vi "Diagnostics Main.vi"() -> ()   [LabVIEW 2015, in "Diagnostics Addon Engine.lvlib"]
uses:
  Diagnostics Addon Engine.lvlib
  Types/Main Configuration.ctl
  Shared/Types/Section Properties.ctl
  Shared/Types/CAN Configuration.ctl
  Shared/Types/CAN Interface.ctl
  Shared/Types/Diagnostic Protocols.ctl
  Shared/Types/Transport Protocols.ctl
  Shared/Types/Security.ctl
  Shared/Types/FPGA Bitfile Settings.ctl
  Shared/Types/Frame Parameters.ctl
  Shared/Types/Signal Parameters.ctl
  Shared/Types/DPID Parameters.ctl
  Shared/Types/DPID Periodic Rate.ctl
  <vilib>/Automotive Diagnostic Command Set/Diagnostic Protocols.llb/DTC Descriptor.ctl
  Types/VS Data Channels.ctl
  SubVIs/Inline Async API/Controls/Write To VS Engine.ctl
  <vilib>/NI Veristand/Custom Device API/Data Reference.ctl
  SubVIs/Inline Async API/Controls/Read From VS Engine.ctl
  <vilib>/NI Veristand/Custom Device API/Block Data Reference.ctl
  SubVIs/Inline Async API/Controls/ReadWrite Data.ctl
  SubVIs/Stop FG/Stop Global Commands.ctl
  SubVIs/Initialize TCP Refs.vi
  STM/RQST Comm_Close All Connections.vi
  SubVIs/Cleanup Conversion Sessions.vi
  STM/RQST Comm Lookup Table_Actions.vi
  <vilib>/Utility/error.llb/Clear Errors.vi
  STM/TCP/STM Get Connection Reference (TCP).vi
  SubVIs/Read GMLAN PIDs and DTCs.vi
  SubVIs/UDS Diagnostics Engine.vi
  <vilib>/NI/Tools/Keyed Array/Add.vi
  <vilib>/NI/AMC/Send Local Message.vi
  <vilib>/NI/AMC/Read Next Message.vi
  STM/TCP Check Connection.vi
  <vilib>/NI/AMC/Send Local Messages.vi
  SubVIs/ScaleAndReplaceAcquiredData.vi
  SubVIs/Initialize Raw XNET Frame.vi
  SubVIs/GMLAN/Utilities/Convert Data to DTCs.vi
  SubVIs/Determine Active DTCs and Timestamps.vi
  SubVIs/Convert Boolean to DBL Array.vi
  SubVIs/GMLAN/_SubVIs/ReadDiagnosticInformation_ByStatus.vi
  SubVIs/GMLAN/_SubVIs/ReadDiagnosticInformation_sendOnChangeDTCCount.vi
  SubVIs/GMLAN/_SubVIs/ReadDiagnosticInformation_readStatusOfDTCByDTCNumber.vi
  SubVIs/GMLAN/_SubVIs/ReadFailureRecordData_readFailureRecordParameters.vi
  SubVIs/GMLAN/GMLAN DynamicallyDefineMessage.vi
  SubVIs/GMLAN/GMLAN ReadDataByPacketIdentifier.vi
  SubVIs/GMLAN/GMLAN InitiateDiagnosticOperation.vi
  SubVIs/GMLAN/GMLAN DisableNormalCommunication.vi
  SubVIs/GMLAN/GMLAN ReturnToNormalMode.vi
  SubVIs/Unlock ECU Security.vi
  <vilib>/NI/Tools/Keyed Array/Index.vi
  SubVIs/GMLAN/GMLAN ClearDiagnosticInformation.vi
  SubVIs/GMLAN/GMLAN DeviceControl.vi
  SubVIs/IndexAndScaleGeneratedData.vi
  SubVIs/GMLAN/GMLAN ReadDataByParameterIdentifier.vi
  SubVIs/Read PIDDIDs.vi
  SubVIs/Tester Present.vi
  <vilib>/NI/Tools/Keyed Array/Map String.vi
  <vilib>/NI/AMC/Create Single Message.vi
  <vilib>/NI/AMC/Update Message Routing Info.vi
  <vilib>/NI/AMC/Read Termination Message.vi
  <vilib>/NI/AMC/Create Multiple Messages.vi
  SubVIs/GMLAN/Utilities/Convert Raw Data to DTCs.vi
  SubVIs/GMLAN/Utilities/GMLAN Service Broadcast.vi
  SubVIs/Execute Security DLL.vi
  SubVIs/GMLAN/GMLAN SecurityAccess.vi
  SubVIs/GMLAN/_SubVIs/SecurityAccess_sendKey.vi
  SubVIs/GMLAN/_SubVIs/SecurityAccess_requestSeed.vi
  SubVIs/GMLAN/GMLAN ReadDataByIdentifier.vi
  SubVIs/GMLAN/GMLAN TesterPresent.vi
  <vilib>/NI/Tools/String/Get Case Matching.vi
  <vilib>/NI/AMC/Destroy Message Queue.vi
  <vilib>/Automotive Diagnostic Command Set/Diagnostic Transport.llb/Close Diagnostic.vi
  <vilib>/xnet/xnet.llb/XNET Database Close.vi
  <vilib>/xnet/xnet.llb/XNET Database Close (Database).vi
  <vilib>/xnet/xnet.llb/XNET Database Delete Object.vi
  <vilib>/xnet/xnet.llb/XNET Database Delete (Cluster).vi
  <vilib>/xnet/xnet.llb/XNET Clear.vi
  Shared/SubVIs/GUID Lookup.vi
  STM/Clear Specific Error.vi
  STM/STM Read Meta Data.vi
  STM/TCP/STM Read Meta Data (TCP Ref).vi
  <vilib>/NI/AMC/Send Message.vi
  <vilib>/Automotive Diagnostic Command Set/Diagnostic Protocols.llb/Convert to Phys.vi
  <vilib>/xnet/xnet.llb/XNET Convert.vi
  <vilib>/xnet/xnet.llb/XNET Convert (Frame Raw to Signal).vi
  SubVIs/Convert ID to Raw Data.vi
  <vilib>/xnet/xnet.llb/XNET Read.vi
  <vilib>/xnet/xnet.llb/XNET Read (Frame CAN).vi
  <vilib>/NI/AMC/Globals.vi
  <vilib>/Automotive Diagnostic Command Set/Diagnostic Protocols.llb/UDS TesterPresent.vi
  <vilib>/Automotive Diagnostic Command Set/Diagnostic Transport.llb/Apply Success Failure Error.vi
  <vilib>/Automotive Diagnostic Command Set/Diagnostic Transport.llb/Diagnostic Service.vi
  <vilib>/Automotive Diagnostic Command Set/Diagnostic Transport.llb/Apply Diagnostic Error.vi
  <vilib>/Automotive Diagnostic Command Set/Diagnostic Transport.llb/Diagnostic Response Recv.vi
  <vilib>/Automotive Diagnostic Command Set/Diagnostic Transport.llb/Diagnostic Service Send.vi
  <vilib>/Automotive Diagnostic Command Set/Diagnostic Transport.llb/Diag Globals.vi
  <vilib>/Automotive Diagnostic Command Set/Diagnostic Protocols.llb/TesterPresent.vi
  <vilib>/Automotive Diagnostic Command Set/Diagnostic Protocols.llb/UDS RoutineControl.vi
  <vilib>/Automotive Diagnostic Command Set/Diagnostic Protocols.llb/StopRoutineByLocalIdentifier.vi
  <vilib>/xnet/xnet.llb/XNET Convert (Signal to Frame Raw).vi
  <vilib>/Automotive Diagnostic Command Set/Diagnostic Protocols.llb/RequestRoutineResultsByLocalIdentifier.vi
  <vilib>/Automotive Diagnostic Command Set/Diagnostic Protocols.llb/StartRoutineByLocalIdentifier.vi
  <vilib>/Automotive Diagnostic Command Set/Diagnostic Protocols.llb/UDS InputOutputControlByIdentifier.vi
  <vilib>/Automotive Diagnostic Command Set/Diagnostic Protocols.llb/InputOutputControlByLocalIdentifier.vi
  <vilib>/Automotive Diagnostic Command Set/Diagnostic Protocols.llb/UDS WriteDataByIdentifier.vi
  <vilib>/Automotive Diagnostic Command Set/Diagnostic Protocols.llb/WriteMemoryByAddress.vi
  <vilib>/Automotive Diagnostic Command Set/Diagnostic Protocols.llb/UDS ReadDataByIdentifier.vi
  <vilib>/Automotive Diagnostic Command Set/Diagnostic Protocols.llb/ReadMemoryByAddress.vi
  <vilib>/Automotive Diagnostic Command Set/Diagnostic Protocols.llb/UDS ECUReset.vi
  <vilib>/Automotive Diagnostic Command Set/Diagnostic Protocols.llb/ECUReset.vi
  <vilib>/Automotive Diagnostic Command Set/Diagnostic Protocols.llb/ReadDataByLocalIdentifier.vi
  <vilib>/Automotive Diagnostic Command Set/Diagnostic Protocols.llb/WriteDataByLocalIdentifier.vi
  <vilib>/Automotive Diagnostic Command Set/Diagnostic Protocols.llb/UDS ClearDiagnosticInformation.vi
  <vilib>/Automotive Diagnostic Command Set/Diagnostic Protocols.llb/ClearDiagnosticInformation.vi
  <vilib>/Automotive Diagnostic Command Set/Diagnostic Protocols.llb/ControlDTCSetting.vi
  <vilib>/Automotive Diagnostic Command Set/Diagnostic Protocols.llb/UDS ControlDTCSetting.vi
  <vilib>/Automotive Diagnostic Command Set/Diagnostic Protocols.llb/ReadDTCByStatus.vi
  <vilib>/Automotive Diagnostic Command Set/Diagnostic Protocols.llb/ReadStatusOfDTC.vi
  <vilib>/Automotive Diagnostic Command Set/Diagnostic Protocols.llb/UDS ReportDTCByStatusMask.vi
  <vilib>/Automotive Diagnostic Command Set/Diagnostic Protocols.llb/UDS ReportSeverityInformationOfDTC.vi
  <vilib>/Automotive Diagnostic Command Set/Diagnostic Protocols.llb/UDS ReportDTCBySeverityMaskRecord.vi
  <vilib>/Automotive Diagnostic Command Set/Diagnostic Protocols.llb/SendKey.vi
  <vilib>/Automotive Diagnostic Command Set/Diagnostic Protocols.llb/UDS SendKey.vi
  <vilib>/Automotive Diagnostic Command Set/Diagnostic Protocols.llb/RequestSeed.vi
  <vilib>/Automotive Diagnostic Command Set/Diagnostic Protocols.llb/UDS RequestSeed.vi
  <vilib>/Automotive Diagnostic Command Set/Diagnostic Protocols.llb/EnableNormalMessageTransmission.vi
  <vilib>/Automotive Diagnostic Command Set/Diagnostic Protocols.llb/UDS CommunicationControl.vi
  <vilib>/Automotive Diagnostic Command Set/Diagnostic Protocols.llb/DisableNormalMessageTransmission.vi
  <vilib>/Automotive Diagnostic Command Set/Diagnostic Protocols.llb/UDS DiagnosticSessionControl.vi
  <vilib>/Automotive Diagnostic Command Set/Diagnostic Protocols.llb/StopDiagnosticSession.vi
  <vilib>/Automotive Diagnostic Command Set/Diagnostic Protocols.llb/StartDiagnosticSession.vi
  <vilib>/Automotive Diagnostic Command Set/Diagnostic Transport.llb/Diag Set Property.vi
  <vilib>/Automotive Diagnostic Command Set/Diagnostic Transport.llb/Diag Get Property.vi
  SubVIs/Sort DPID IDs by Speed.vi
  STM/TCP/STM Write Message (TCP).vi
  <vilib>/NI/AMC/Create Message Queue.vi
  STM/TCP/STM Read Message (TCP).vi
  SubVIs/Stop FG/Initialize Global Stop.vi
  SubVIs/Initialize CAN.vi
  STM/RQST Comm Lookup Table_Initialize.vi
  SubVIs/Stop FG/Stop FG.lvlib
  <vilib>/NI Veristand/Custom Device Tools/Custom Device Utility Library/Custom Device Utility Library.lvlib
  SubVIs/Inline Async API/Inline Async API.lvlib
  SubVIs/Error Handling API/Error Handling API.lvlib
  <vilib>/Utility/error.llb/DialogType.ctl
  Shared/Diagnostics Addon Shared.lvlib
  <vilib>/NI Veristand/Custom Device API/Custom Device API.lvlib
panel:
  in  "Parameters":T1={"Properties"={"Name"="", "CAN"={"Database File"=path "", "CAN Interface"=enum."CAN0", "Baud Rate"=0, "Diagnostic Protocol"=enum."GMLAN", "Transport Protocol"=enum."ISO TP - Normal Mode", "Transmit ID"=0, "Receive ID"=0, "Transmit Extension"=0, "Receive Extension"=0, "Receive UUDT ID"=0, "Enable Stream"=TRUE, "VW TP Channel ID"=0, "Security"={"Source DLL Path"=path "", "Security Level"=1, "Target DLL Path"=path ""}, "Fill Frame"=FALSE, "Fill Byte"=255, "Termination"=FALSE}, "FPGA Settings"={"RT Bitfile Path"=path "", "RIO Device"=0, "Enable"=FALSE}, "PIDs"=[], "PID Lookup"=variant, "CPIDs"=[], "CPID Lookup"=variant, "DIDs"=[], "DID Lookup"=variant, "DPIDs"=[], "DPID Lookup"=variant, "DTC descriptor"={"DTC Byte Length"=2, "Status Byte Length"=1, "Add Data Byte Length"=1, "Byte Order"=enum."Motorola"}, "Routine.Start.Cmd Lookup"=variant, "Routine.Status.Cmd Lookup"=variant, "Routine.Stop.Cmd Lookup"=variant, "IO.Cmd Lookup"=variant, "IO.Resp Lookup"=variant, "Routine.Start.Resp Lookup"=variant, "Routine.Status.Resp Lookup"=variant, "Routine.Stop.Resp Lookup"=variant, "Memory.Write Lookup"=variant, "Memory.Read Lookup"=variant}, "ChanRefs"={"ToVS.PIDs"={"Name"="", "Write to VS Engine FIFO"=refnum, "Pairs"={"Refs"=[], "Values"=[]}}, "ToVS.DIDs"={"Name"="", "Write to VS Engine FIFO"=refnum, "Pairs"={"Refs"=[], "Values"=[]}}, "ToVS.DTCs"={"Name"="", "Write to VS Engine FIFO"=refnum, "Pairs"={"Refs"=[], "Values"=[]}}, "ToVS.DTCCount"={"Name"="", "Write to VS Engine FIFO"=refnum, "Pairs"={"Refs"=[], "Values"=[]}}, "ToVS.Status"={"Name"="", "Write to VS Engine FIFO"=refnum, "Pairs"={"Refs"=[], "Values"=[]}}, "FromVS.CPIDs"={"Name"="", "Read from VS Engine FIFO"=refnum, "Pairs"={"Refs"=[], "Values"=[]}}, "Cmds"={"Name"="", "Write to VS Engine FIFO"=refnum, "Read from VS Engine FIFO"=refnum, "Pairs"={"Chan Refs"=[], "Prev. Values"=[]}}, "ToVS.Routine.Start"={"Name"="", "Write to VS Engine FIFO"=refnum, "Pairs"={"Refs"=[], "Values"=[]}}, "FromVS.Routine.Start"={"Name"="", "Read from VS Engine FIFO"=refnum, "Pairs"={"Refs"=[], "Values"=[]}}, "ToVS.Routine.Stop"={"Name"="", "Write to VS Engine FIFO"=refnum, "Pairs"={"Refs"=[], "Values"=[]}}, "FromVS.Routine.Stop"={"Name"="", "Read from VS Engine FIFO"=refnum, "Pairs"={"Refs"=[], "Values"=[]}}, "ToVS.Routine.Status"={"Name"="", "Write to VS Engine FIFO"=refnum, "Pairs"={"Refs"=[], "Values"=[]}}, "FromVS.Routine.Status"={"Name"="", "Read from VS Engine FIFO"=refnum, "Pairs"={"Refs"=[], "Values"=[]}}, "FromVS.IO.Cmd"={"Name"="", "Read from VS Engine FIFO"=refnum, "Pairs"={"Refs"=[], "Values"=[]}}, "ToVS.IO.Resp"={"Name"="", "Write to VS Engine FIFO"=refnum, "Pairs"={"Refs"=[], "Values"=[]}}, "FromVS.WriteMemory"={"Name"="", "Read from VS Engine FIFO"=refnum, "Pairs"={"Refs"=[], "Values"=[]}}, "ToVS.ReadMemory"={"Name"="", "Write to VS Engine FIFO"=refnum, "Pairs"={"Refs"=[], "Values"=[]}}}} {"ChanRefs"."ToVS.ReadMemory"."Pairs"."Refs" format="%.0x"; "ChanRefs"."FromVS.WriteMemory"."Pairs"."Refs"."Data Reference" format="%.0x"; "ChanRefs"."ToVS.IO.Resp"."Pairs"."Refs" format="%.0x"; "ChanRefs"."FromVS.IO.Cmd"."Pairs"."Refs"."Data Reference" format="%.0x"; "ChanRefs"."FromVS.Routine.Status"."Pairs"."Refs"."Data Reference" format="%.0x"; "ChanRefs"."ToVS.Routine.Status"."Pairs"."Refs" format="%.0x"; "ChanRefs"."FromVS.Routine.Stop"."Pairs"."Refs"."Data Reference" format="%.0x"; "ChanRefs"."ToVS.Routine.Stop"."Pairs"."Refs" format="%.0x"; "ChanRefs"."FromVS.Routine.Start"."Pairs"."Refs"."Data Reference" format="%.0x"; "ChanRefs"."ToVS.Routine.Start"."Pairs"."Refs" format="%.0x"; "ChanRefs"."Cmds"."Pairs"."Chan Refs" format="%.0x"; "ChanRefs"."FromVS.CPIDs"."Pairs"."Refs"."Data Reference" format="%.0x"; "ChanRefs"."ToVS.Status"."Pairs"."Refs" format="%.0x"; "ChanRefs"."ToVS.DTCCount"."Pairs"."Refs" format="%.0x"; "ChanRefs"."ToVS.DTCs"."Pairs"."Refs" format="%.0x"; "ChanRefs"."ToVS.PIDs"."Pairs"."Refs" format="%.0x"; "ChanRefs"."ToVS.DIDs"."Pairs"."Refs" format="%.0x"; "Properties"."CPIDs"."Signals"."Byte Order" items=["Little Endian", "Big Endian"]; "Properties"."CPIDs"."Signals"."Data Type" items=["Signed", "Unsigned", "IEEE Float"]; "Properties"."DIDs"."Signals"."Byte Order" items=["Little Endian", "Big Endian"]; "Properties"."DIDs"."Signals"."Data Type" items=["Signed", "Unsigned", "IEEE Float"]; "Properties"."CAN"."Fill Byte" format="%.0x"; "Properties"."CAN"."VW TP Channel ID" format="%.0x"; "Properties"."CAN"."Receive UUDT ID" format="%.0x"; "Properties"."CAN"."Receive Extension" format="%.0x"; "Properties"."CAN"."Transmit Extension" format="%.0x"; "Properties"."CAN"."Receive ID" format="%.0x"; "Properties"."CAN"."Transmit ID" format="%.0x"; "Properties"."PIDs"."Signals"."Byte Order" items=["Little Endian", "Big Endian"]; "Properties"."PIDs"."Signals"."Data Type" items=["Signed", "Unsigned", "IEEE Float"]}
  in  "Error":errorcluster
  in  "Parent":string
  in  "stop":bool
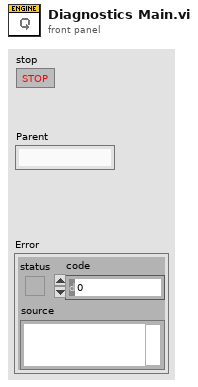
[diagram p1: front panel]
types:
  T1 = typedef "Diagnostics Addon Engine.lvlib/Main Configuration.ctl" = cluster{"Properties":T2, "ChanRefs":T14}
  T2 = typedef "Diagnostics Addon Shared.lvlib/Section Properties.ctl" = cluster{"Name":string, "CAN":T3, "FPGA Settings":T8, "PIDs":T9[], "PID Lookup":variant, "CPIDs":T9[], "CPID Lookup":variant, "DIDs":T9[], "DID Lookup":variant, "DPIDs":T11[], "DPID Lookup":variant, "DTC descriptor":T13, "Routine.Start.Cmd Lookup":variant, "Routine.Status.Cmd Lookup":variant, "Routine.Stop.Cmd Lookup":variant, "IO.Cmd Lookup":variant, "IO.Resp Lookup":variant, "Routine.Start.Resp Lookup":variant, "Routine.Status.Resp Lookup":variant, "Routine.Stop.Resp Lookup":variant, "Memory.Write Lookup":variant, "Memory.Read Lookup":variant}
  T3 = typedef "Diagnostics Addon Shared.lvlib/CAN Configuration.ctl" = cluster{"Database File":path, "CAN Interface":T4, "Baud Rate":u32, "Diagnostic Protocol":T5, "Transport Protocol":T6, "Transmit ID":u32, "Receive ID":u32, "Transmit Extension":u8, "Receive Extension":u8, "Receive UUDT ID":u32, "Enable Stream":bool, "VW TP Channel ID":u32, "Security":T7, "Fill Frame":bool, "Fill Byte":u8, "Termination":bool}
  T4 = typedef "Diagnostics Addon Shared.lvlib/CAN Interface.ctl" = enum16{"CAN0", "CAN1", "CAN2", "CAN3", "CAN4", "CAN5", "CAN6", "CAN7", "CAN8", "CAN9", "CAN10", "CAN11", "CAN12", "CAN13", "CAN14", "CAN15", "CAN16", "CAN17", "CAN18", "CAN19", "CAN20", "CAN21", "CAN22", "CAN23", "CAN24", "CAN25", "CAN26", "CAN27", "CAN28", "CAN29", "CAN30", "CAN31", "CAN32", "CAN33", "CAN34", "CAN35", "CAN36", "CAN37", "CAN38", "CAN39", "CAN40", "CAN41", "CAN42", "CAN43", "CAN44", "CAN45", "CAN46", "CAN47", "CAN48", "CAN49", "CAN50", "CAN51", "CAN52", "CAN53", "CAN54", "CAN55", "CAN56", "CAN57", "CAN58", "CAN59", "CAN60", "CAN61", "CAN62", "CAN63", "CAN 256 (Virtual)", "CAN 257 (Virtual)"}
  T5 = typedef "Diagnostics Addon Shared.lvlib/Diagnostic Protocols.ctl" = enum16{"GMLAN", "KWP-2000", "UDS"}
  T6 = typedef "Diagnostics Addon Shared.lvlib/Transport Protocols.ctl" = enum16{"ISO TP - Normal Mode", "ISO TP - Mixed Mode", "VW TP 2.0", "Diagnostics on IP"}
  T7 = typedef "Diagnostics Addon Shared.lvlib/Security.ctl" = cluster{"Source DLL Path":path, "Security Level":u8, "Target DLL Path":path}
  T8 = typedef "Diagnostics Addon Shared.lvlib/FPGA Bitfile Settings.ctl" = cluster{"RT Bitfile Path":path, "RIO Device":u16, "Enable":bool}
  T9 = typedef "Diagnostics Addon Shared.lvlib/Frame Parameters.ctl" = cluster{"Name":string, "Description":string, "ID":u16, "Signals":T10[]}
  T10 = typedef "Diagnostics Addon Shared.lvlib/Signal Parameters.ctl" = cluster{"Start Bit":u8, "Length":u8, "Scaling Factor":dbl, "Scaling Offset":dbl, "Minimum":dbl, "Maximum":dbl, "Data Type":u32, "Byte Order":u32, "Default Value":dbl, "Name":string, "Units":string, "Description":string}
  T11 = typedef "Diagnostics Addon Shared.lvlib/DPID Parameters.ctl" = cluster{"DPID ID":u8, "Speed":T12, "PIDs":u16[]}
  T12 = typedef "Diagnostics Addon Shared.lvlib/DPID Periodic Rate.ctl" = enum16{"Slow", "Medium", "Fast"}
  T13 = typedef "Diagnostics Addon Shared.lvlib/DTC Descriptor.ctl" = cluster{"DTC Byte Length":i32, "Status Byte Length":i32, "Add Data Byte Length":i32, "Byte Order":enum16{"Motorola", "Intel"}}
  T14 = typedef "Diagnostics Addon Engine.lvlib/VS Data Channels.ctl" = cluster{"ToVS.PIDs":T15, "ToVS.DIDs":T15, "ToVS.DTCs":T15, "ToVS.DTCCount":T15, "ToVS.Status":T15, "FromVS.CPIDs":T17, "Cmds":T19, "ToVS.Routine.Start":T15, "FromVS.Routine.Start":T17, "ToVS.Routine.Stop":T15, "FromVS.Routine.Stop":T17, "ToVS.Routine.Status":T15, "FromVS.Routine.Status":T17, "FromVS.IO.Cmd":T17, "ToVS.IO.Resp":T15, "FromVS.WriteMemory":T17, "ToVS.ReadMemory":T15}
  T15 = typedef "Diagnostics Addon Engine.lvlib/Inline Async API.lvlib/Write To VS Engine.ctl" = cluster{"Name":string, "Write to VS Engine FIFO":refnum<k33>, "Pairs":cluster{"Refs":T16[], "Values":dbl[]}}
  T16 = typedef "Custom Device API.lvlib/Data Reference.ctl" = i32
  T17 = typedef "Diagnostics Addon Engine.lvlib/Inline Async API.lvlib/Read From VS Engine.ctl" = cluster{"Name":string, "Read from VS Engine FIFO":refnum<k33>, "Pairs":cluster{"Refs":T18[], "Values":dbl[]}}
  T18 = typedef "Custom Device API.lvlib/Block Data Reference.ctl" = cluster{"Data Reference":T16, "Offset":u64, "Length":u64}
  T19 = typedef "Diagnostics Addon Engine.lvlib/Inline Async API.lvlib/ReadWrite Data.ctl" = cluster{"Name":string, "Write to VS Engine FIFO":refnum<k33>, "Read from VS Engine FIFO":refnum<k33>, "Pairs":cluster{"Chan Refs":T16[], "Prev. Values":dbl[]}}
  T20 = typedef "Diagnostics Addon Engine.lvlib/State Variables.ctl" = cluster{"TCP Refs":T21, "Stop":T23, "Top VI":refnum<vi>, "Parameters":T1, "ADCS Connection":T24, "XNET References":T26, "BufferedCmds":T27, "XNETEngine (GMLAN)":T27}
  T21 = typedef "Diagnostics Addon Engine.lvlib/TCP Refs.ctl" = cluster{"Connection List":T22, "listener ID":refnum<k5>}
  T22 = typedef "Diagnostics Addon Engine.lvlib/STM Lookup Table Ref.ctl" = refnum<vi>
  T23 = typedef "Diagnostics Addon Engine.lvlib/Stop FG.lvlib/Stop Global Ref.ctl" = refnum<vi>
  T24 = typedef "NI_Automotive Diagnostic Command Set.lvlib/Diag Reference.ctl" = cluster{"Diag CAN Handle":u32, "Transport Protocol":T25, "Receive Address Extension":u8, "Transmit Address Extension":u8, "Receive CAN Id":u32, "Transmit CAN Id":u32, "Diag CAN Queue":refnum<queue>, "Log Frames ?":bool, "My TP Address":u8, "Other TP Address":u8, "T1":u16, "T2":u16, "T3":u16, "T4":u16, "Tx SN":u8, "Block Size":u8, "Rx SN":u8, "VW TP Initialized?":bool, "Tx block no":u8, "baud rate":u32, "Interface":string, "Channel Diag CAN Handle":u32, "UDP Connection ID":refnum<k16>, "TCP Connection ID":refnum<k5>, "Target IP Addr":u32, "Source Address":u16, "Target Address":u16, "Send Header NACK?":bool, "DLL Handle":u32, "NAD":u8, "Time Stamp read first":dbl, "Time Stamp read last":dbl, "Time Stamp write first":dbl, "Time Stamp write last":dbl, "Time Stamp write":dbl, "Time Stamp read":dbl}
  T25 = typedef "NI_Automotive Diagnostic Command Set.lvlib/Transport Protocol Selector.ctl" = enum16{"ISO TP - Normal Mode", "ISO TP - Mixed Mode", "VW TP 2.0", "Diagnostics on IP", "ISO TP LIN"}
  T26 = typedef "Diagnostics Addon Engine.lvlib/XNET References.ctl" = cluster{"Database":refnum<k21>, "GMLAN DPID Session":refnum<k21>, "Cluster":refnum<k21>}
  T27 = typedef "AMC.lvlib/Message Queue.ctl" = refnum<queue>
  T28 = typedef "Diagnostics Addon Engine.lvlib/Stop FG.lvlib/Stop Global Commands.ctl" = enum16{"Write", "Read", "Reset"}
  T29 = typedef "DialogType.ctl" = u16
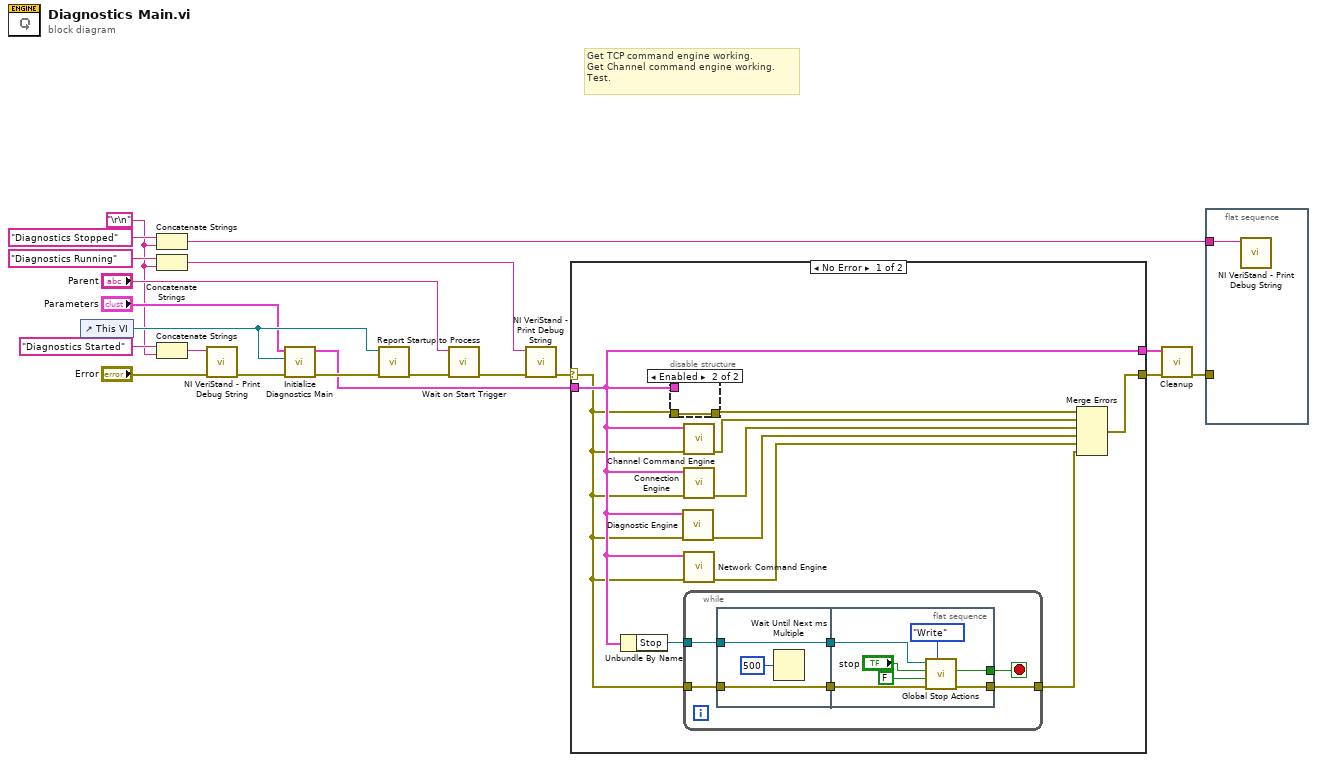
[diagram p0: block diagram]
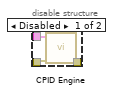
[diagram p2: hidden frame]
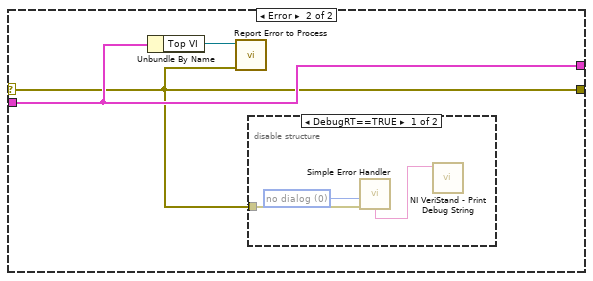
[diagram p3: hidden frame]
diagram:
  w1 = "\r\n"
  # "Get TCP command engine working.\nGet Channel command engine working.\nTest."
  n1 = control-ref of="This VI"() -> (w15:refnum<vi>)
  n2 = Concatenate Strings("Diagnostics Stopped" ("Debug String"), w1) -> (w2:string)
  n3 = Concatenate Strings("Diagnostics Running" ("Debug String"), w1) -> (w4:string)
  n4 = Concatenate Strings("Diagnostics Started" ("Debug String"), w1) -> (w6:string)
  n5 = call <vilib>:"NI VeriStand - Print Debug String.vi"("error in (no error)"="Error", "Message"=w6) -> ("error out"=w14:errorcluster)  [unwired: 9 in]
  n6 = call "Initialize Diagnostics Main.vi"("error in (no error)"=w14, "This VI"=w15, "Parameters"="Parameters") -> ("error out"=w13:errorcluster, "State Variables Out"=w11:T20)  [unwired: 7 in]
  n7 = call "Report Startup to Process.vi"("Error"=w13, "This VI"=w15) -> ("error out"=w16:errorcluster)  [unwired: 9 in]
  n8 = call "Wait on Start Trigger.vi"("error in (no error)"=w16, "Name"="Parent") -> ("error out"=w17:errorcluster)  [unwired: 8 in, 1 out]
  n9 = call <vilib>:"NI VeriStand - Print Debug String.vi"("error in (no error)"=w17, "Message"=w4) -> ("error out"=w9:errorcluster)  [unwired: 9 in]
  n10 = case shown="No Error" w9 {
    selector: w9 -> [w22 w51]
    tunnel: [w30 w51] -> w12
    tunnel: w11 -> [w23 w53]
    tunnel: [w23 w53] -> w8
    frame No Error {
      n11 = Unbundle By Name(w23) -> ("Stop"=w29:T23)
      n12 = disable-structure shown="Enabled" {
        disable-tunnel: w23 -> [w33 _]
        disable-tunnel: w22 -> [w32 w34]
        disable-tunnel: [w31 w34] -> w21
        frame Disabled {
          n13 = call "CPID Engine.vi"("error in"=w32, "State Variables"=w33) -> ("error out"=w31:errorcluster)  [unwired: 9 in]
        }
        frame Enabled {
        }
      }
      n14 = call "Diagnostic Engine.vi"("error in (no error)"=w22, "State Variables"=w23) -> ("error out"=w27:errorcluster)  [unwired: 9 in]
      n15 = call "Channel Command Engine.vi"("error in"=w22, "State Variables"=w23) -> ("error out"=w24:errorcluster)  [unwired: 9 in]
      n16 = call "Connection Engine.vi"("error in (no error)"=w22, "State Variables"=w23) -> ("error out"=w28:errorcluster)  [unwired: 9 in]
      n17 = call "Network Command Engine.vi"("error in (no error)"=w22, "State Variables"=w23) -> ("error out"=w25:errorcluster)  [unwired: 9 in]
      n18 = while {
        tunnel: w22 -> [w40]
        tunnel: w29 -> [w38]
        tunnel: [w35] -> w26
        stop <- w39 stop-if-true
        n19 = flat-sequence {
          tunnel: w38 -> [w42]
          tunnel: w40 -> [w43]
          tunnel: [w43] -> w37
          tunnel: [w42] -> w36
          tunnel: [w47] -> w35
          tunnel: [w45] -> w39
          tunnel: w37 -> [w48]
          tunnel: w36 -> [w44]
          frame #0 {
            n20 = Wait Until Next ms Multiple(millisecond multiple=u32 500) -> ()  [unwired: 1 out]
          }
          frame #1 {
            n21 = call "Global Stop Actions.vi"("Command"=Stop_Global_Commands."Write", "error in (no error)"=w48, "Stop on Error?"=FALSE, "Stop?"="stop", "vi reference"=w44) -> ("error out"=w47:errorcluster, "Latched Stop"=w45:bool)  [unwired: 4 in, 1 out]
          }
        }
      }
      n22 = Merge Errors(w21, w24, w28, w27, w25, w26) -> (w30:errorcluster)
    }
    frame Error {
      n23 = Unbundle By Name(w53) -> ("Top VI"=w52:refnum<vi>)
      n24 = call "Report Error to Process.vi"("Error"=w51, "This VI"=w52) -> ()  [unwired: 10 in]
      n25 = disable-structure shown="DebugRT==TRUE" {
        disable-tunnel: w51 -> [w56 _]
        frame condition #0 {
          w55 = T29 0 items=["no dialog", "OK message", "continue or stop message", "OK message + warnings", "continue/stop + warnings"] ("type of dialog (OK msg:1)")
          n26 = call <vilib>:"Simple Error Handler.vi"("type of dialog (OK msg:1)"=w55, "error in (no error)"=w56) -> ("message"=w54:string)  [unwired: 3 in, 4 out]
          n27 = call <vilib>:"NI VeriStand - Print Debug String.vi"("Message"=w54) -> ()  [unwired: 10 in, 1 out]
        }
        frame condition #1 (active) {
        }
      }
    }
  }
  n28 = call "Cleanup.vi"("error in (no error)"=w12, "State Variables"=w8) -> ("error out"=w10:errorcluster)  [unwired: 9 in]
  n29 = flat-sequence {
    tunnel: w10 -> [_]
    tunnel: w2 -> [w57]
    frame #0 {
      n30 = call <vilib>:"NI VeriStand - Print Debug String.vi"("Message"=w57) -> ()  [unwired: 10 in, 1 out]
    }
  }
